vi "Digit to color converter.vi"(4 "Digit":T1) -> (1 "Digit color":u32(colorbox))   [LabVIEW 2018, in "Enum to Color Converter.lvlib"]
uses:
  Digit--control.ctl
  Enum to Color Converter.lvlib
  Resistor Band Colors/Resistor Band Colors.lvlib
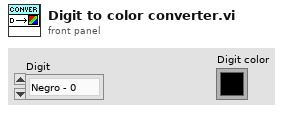
[diagram p1: front panel]
types:
  T1 = typedef "Digit--control.ctl" = enum16{"Negro - 0", "Marron - 1", "Rojo - 2", "Naranja - 3", "Amarillo - 4", "Verde - 5", "Azul - 6", "Violeta - 7", "Gris - 8", "Blanco - 9"}
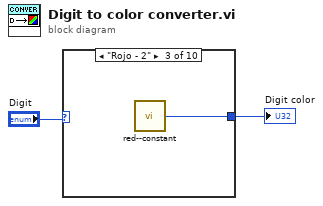
[diagram p0: block diagram]
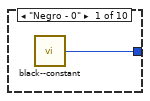
[diagram p2: hidden frame]
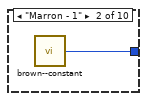
[diagram p3: hidden frame]
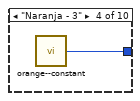
[diagram p4: hidden frame]
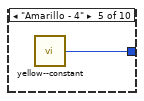
[diagram p5: hidden frame]
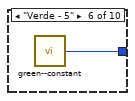
[diagram p6: hidden frame]
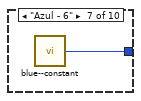
[diagram p7: hidden frame]
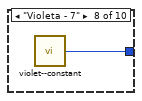
[diagram p8: hidden frame]
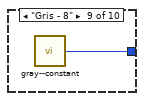
[diagram p9: hidden frame]
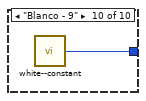
[diagram p10: hidden frame]
diagram:
  n1 = case shown="\"Rojo - 2\"" "Digit" {
    tunnel: [w3 w4 w5 w6 w7 w8 w9 w10 w11 w12] -> w1
    frame "Negro - 0" {
      n2 = call "black--constant.vi"() -> ("Negro"=w3:u32)  [unwired: 5 in]
    }
    frame "Marron - 1" {
      n3 = call "brown--constant.vi"() -> ("brown"=w4:u32)  [unwired: 5 in]
    }
    frame "Rojo - 2" {
      n4 = call "red--constant.vi"() -> ("red"=w5:u32)  [unwired: 5 in]
    }
    frame "Naranja - 3" {
      n5 = call "orange--constant.vi"() -> ("orange"=w6:u32)  [unwired: 5 in]
    }
    frame "Amarillo - 4" {
      n6 = call "yellow--constant.vi"() -> ("yellow"=w7:u32)  [unwired: 5 in]
    }
    frame "Verde - 5" {
      n7 = call "green--constant.vi"() -> ("green"=w8:u32)  [unwired: 5 in]
    }
    frame "Azul - 6" {
      n8 = call "blue--constant.vi"() -> ("blue"=w9:u32)  [unwired: 5 in]
    }
    frame "Violeta - 7" {
      n9 = call "violet--constant.vi"() -> ("violet"=w10:u32)  [unwired: 5 in]
    }
    frame "Gris - 8" {
      n10 = call "gray--constant.vi"() -> ("gray"=w11:u32)  [unwired: 5 in]
    }
    frame "Blanco - 9" {
      n11 = call "white--constant.vi"() -> ("white"=w12:u32)  [unwired: 5 in]
    }
  }
  "Digit color" <- w1
